vi "Count N Points (SubVI).vi"(7 "N Points":u16, 11 "Count In":u16) -> (3 "Count Out":u16)   [LabVIEW 2015]
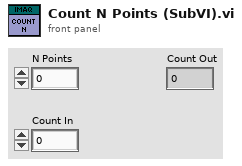
[diagram p1: front panel]
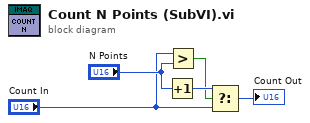
[diagram p0: block diagram]
diagram:
  n1 = Increment(x="N Points") -> (x+1=w4:u16)
  n2 = Greater?(x="Count In", y="N Points") -> (0:w1:bool)
  n3 = Select(t=w4, s=w1, f="Count In") -> (s? t:f=→"Count Out":u16)
